vi "Check Slices Done.vi"(9 "Slices Done":u16, 11 "Total Number of Slices":u16) -> (1 "Slices Done":u16, 3 "Stack Done":bool=TRUE)   [LabVIEW 2014]
panel:
  # "Copyright 2014 Vidrio Technologies\nScanImage 5 software is licensed under the Apache License, Version 2.0 (the \"License\"); you may not use any files contained\nwithin the ScanImage 5 release except in compliance with the License. You may obtain a copy of the License at\n http://www.apache.org/licenses/LICENSE-2.0\nUnless required by applicable law or agreed to in writing, software distributed under the License is distributed on an\n\"AS IS\" BASIS, WITHOUT WARRANTIES OR CONDITIONS OF ANY KIND, either express or implied. See the License for the\n specific language governing permissions and limitations under the License."
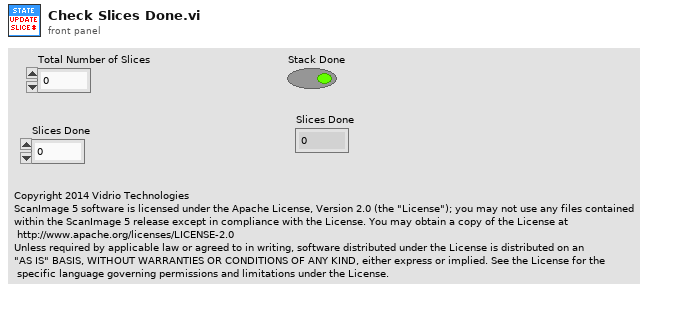
[diagram p1: front panel]
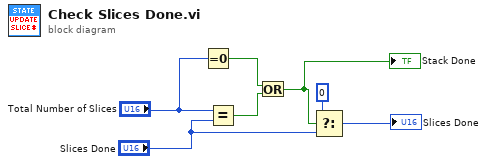
[diagram p0: block diagram]
diagram:
  n1 = Equal To 0?(x="Total Number of Slices") -> (x = 0?=w6:bool)
  n2 = Equal?(x="Total Number of Slices", y="Slices Done") -> (x = y?=w5:bool)
  n3 = Or(x=w6, y=w5) -> (x .or. y?=w1:bool)
  "Stack Done" <- w1
  n4 = Select(t=u16 0, s=w1, f="Slices Done") -> (s? t:f=→"Slices Done":u16)
